vi "Create Events.vi"(8 "error in (no error)":errorcluster, 11 "CIF_UI in":refnum<class "CIF_UI.lvclass">) -> (0 "error out":errorcluster, 3 "CIF_UI out":refnum<class "CIF_UI.lvclass">)   [LabVIEW 2021, in "CIF_UI.lvclass"]
uses:
  CIF_UI.lvclass
  Typedef/New Connection Plugin Event Data.ctl
  Typedef/New Connection Event Data.ctl
  <vilib>/gRPC/LabVIEW gRPC Library/Shared/grpcId.ctl
  CIF_UI.lvclass/CIF_UI.ctl
  <vilib>/gRPC/LabVIEW gRPC Library/grpc-lvsupport-release.lvlib
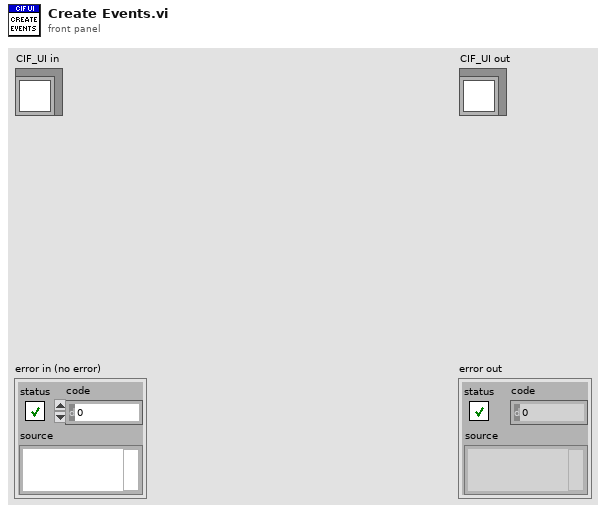
[diagram p1: front panel]
types:
  T1 = typedef "CIF_UI.lvclass/New Connection Plugin Event Data.ctl" = cluster{"IP Address and Port":string, "Connected":bool}
  T2 = typedef "CIF_UI.lvclass/New Connection Event Data.ctl" = cluster{"Manager gRPC ID":T3, "IP Address":string, "Connected":bool}
  T3 = typedef "grpc-lvsupport-release.lvlib/grpcId.ctl" = u64
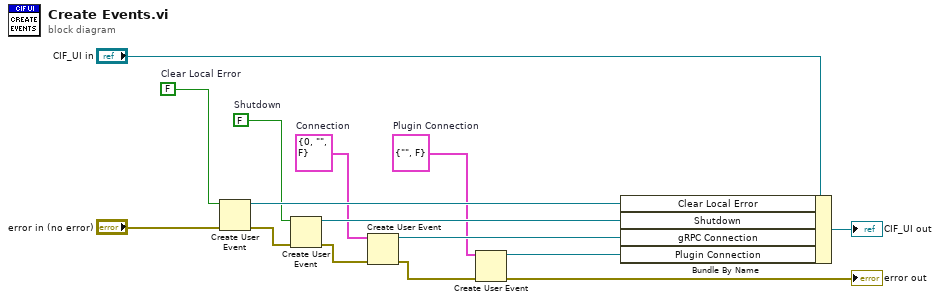
[diagram p0: block diagram]
diagram:
  w5 = T1 {"IP Address and Port"="", "Connected"=FALSE}  # Plugin Connection
  w6 = T2 {"Manager gRPC ID"=0, "IP Address"="", "Connected"=FALSE}  # Connection
  w11 = FALSE  # Shutdown
  w13 = FALSE  # Clear Local Error
  n1 = Create User Event(user event datatype=w13, error in="error in (no error)") -> (user event=w12:refnum<user-event>, error out=w10:errorcluster)
  n2 = Create User Event(user event datatype=w11, error in=w10) -> (user event=w8:refnum<user-event>, error out=w9:errorcluster)
  n3 = Create User Event(user event datatype=w6, error in=w9) -> (user event=w7:refnum<user-event>, error out=w3:errorcluster)
  n4 = Create User Event(user event datatype=w5, error in=w3) -> (user event=w1:refnum<user-event>, error out=→"error out":errorcluster)
  n5 = Bundle By Name(cluster="CIF_UI in", "Clear Local Error"=w12, "Shutdown"=w8, "gRPC Connection"=w7, "Plugin Connection"=w1) -> (→"CIF_UI out":refnum<class "CIF_UI.lvclass">)
